vi "ADC SNR_ref_sweep.vi"(8 "error in (no error)":errorcluster, 9 "Sequence parameters":string[][](array[string])=[["Min limit", "Max limit", "Register sheet file", "Register Sheet"], ["", "", "CC2600.xls", "TX_BLE;Trim"], ["Reg write (addr;value)", "Operating frequency [Hz]", "", ""], ["NA", "2.44G", "", ""]], 10 "Run type":i32, 11 "Method parameters":T3={"Dev"={"Do not disturb DUT"=FALSE, "XOSC"=32000000.0, "Board type"="", "EM"="", "Configure tempboard"=TRUE, "Device specific info"=[], "Generic Object"=refnum}, "Method"={"Run type"=1, "Test name"="Current LPM2 4", "Comment"="", "Results folder"="", "AFC"=enum."Off", "Method name"="Current LPM2 4", "Method results"={"Excel brief report"=FALSE, "Spotfire report"=FALSE, "Starfish report"=FALSE}, "Operator"="", "Reference time"=timestamp(0 s since 1904-01-01), "AFC delay"=0.0, "Initialization"=enum."Enabled", "MD5 Sum"="", "HW addon board"=enum."None", "AFC Regsheet"="", "AFC Regfile"=path "", "dummy"=0.0}, "Inst"={"Instr"={"PS1"={"Name"="", "GPIB address"="", "VISA session"=""}, "PS2"={"Name"="", "GPIB address"="", "VISA session"=""}, "TC1"={"Name"="", "GPIB address"="", "VISA session"=""}, "TC2"={"Name"="", "GPIB address"="", "VISA session"=""}, "SA1"={"Name"="", "GPIB address"="", "VISA session"=""}, "SA2"={"Name"="", "GPIB address"="", "VISA session"=""}, "SG1"={"Name"="", "GPIB address"="", "VISA session"=""}, "SG2"={"Name"="", "GPIB address"="", "VISA session"=""}, "SG3"={"Name"="", "GPIB address"="", "VISA session"=""}, "MI1"={"Name"="", "GPIB address"="", "VISA session"=""}, "MI2"={"Name"="", "GPIB address"="", "VISA session"=""}, "SW SA"={"Name"="", "Controller addr"=""}, "SW SG"={"Name"="", "Controller addr"=""}, "MI3"={"Name"="", "GPIB address"="", "VISA session"=""}}, "Switchbox"={"RF Path"=0, "Cal compensation"=enum."TX", "Switchbox gain mode"="", "State"=enum."TX"}, "Instr to control (i.e. SA1)"="Default", "Intrument info string"=""}, "Sequence parameters"=[["Weight", "Min Limit", "Max Limit", "Register Sheet", "", "", "", "", "", "", "", "", ""], ["Vital", "", "1", "LPM2", "", "", "", "", "", "", "", "", ""], ["Resolution", "Reg write (addr;value)", "Chip mode", "Range", "", "", "", "", "", "", "", "", ""], ["u", "NA", "", "auto", "", "", "", "", "", "", "", "", ""]], "Cond"={"Temp logged"=25.0, "VDD1_PS1_6V"=-999.0, "VDD2_PS1_25V"=-999.0, "VDD4_PS2_25V"=-999.0, "VDD3_PS2_6V"=-999.0}, "Meas config"={"X-axis inner loop index"=32000000, "Y-axis outer loop index"=32000000, "X-axis"=[], "Y-axis"=[], "X-axis array req size"=32000000, "Y-axis array req size"=32000000, "Param description"=[], "Use meas clust for reporting"=FALSE, "Parameter index (page)"=0, "X-axis name"="", "Y-axis name"=""}} {"Cond"."VDD3_PS2_6V" format="%.3f"; "Cond"."VDD4_PS2_25V" format="%.3f"; "Cond"."VDD2_PS1_25V" format="%.3f"; "Cond"."VDD1_PS1_6V" format="%.3f"; "Method"."dummy" format="%.1p"; "Method"."AFC delay" format="%.1p"; "Dev"."XOSC" format="%.3p"}) -> (0 "error out":errorcluster, 1 "End method error":T2, 2 "Short Results":string[](array[string])=["0.00", "0.00", "0.00", "0.00"], 3 "Result summary":string[][](array[string])=[["Critical", "Output Power@2405 MHz", "-3", "4", "dBm"], ["Critical", "Output Power@2410 MHz", "-3", "4", "dBm"]])   [LabVIEW 2019]
doc: "[AutoDocStart]Performs crystal accuracy measurements. Measures the offset from ideal frequency. Primarily used for tuning XOSC capacitors and verifying XOSC trims.\n\nSweeping parameters: operating frequency, OSC override value and VDDR level\n\nResults: Offset frequency in ppm[AutoDocEnd]"
uses:
  User Lib/Utilities/Cluster definitions/Method input.ctl
  User Lib/Utilities/Cluster definitions/Device specific info.ctl
  User Lib/Utilities/Controls/Automatic Frequency Compensation types.ctl
  User Lib/Utilities/Controls/Method Reports.ctl
  User Lib/Utilities/Cluster definitions/Method Initialization.ctl
  User Lib/Utilities/Controls/HW addon boards.ctl
  User Lib/Utilities/Cluster definitions/Instr clust.ctl
  User Lib/Utilities/Switchbox control/SwitchBox_State._ENUMctl.ctl
  User Lib/Utilities/Cluster definitions/End method error cluster.ctl
  User Lib/Utilities/Cluster definitions/DUT vdd control.ctl
  User Lib/Utilities/Cluster definitions/DUT VDD4.ctl
  User Lib/Utilities/Cluster definitions/DUT VDD3.ctl
  User Lib/Utilities/Cluster definitions/DUT VDD2.ctl
  User Lib/Utilities/Cluster definitions/DUT VDD1.ctl
  3a26386c-adf8-4bfd-9313-23d3b8777f38.vi
  00a85a70-9fe7-4572-b3d9-e5ce3378243e.vi
  50564926-5797-4515-82f7-8b24a758fedb.vi
  ff8123cc-dee3-4505-8a81-37fe2d556b47.vi
  fd6c0d4b-9dc8-492c-9bac-41f6ad4bdd39.vi
  153c9ed0-a16e-46e5-8e4c-c1ec3d6952ee.vi
  ce3ff4de-b0d2-4c44-a033-17b5da13a9db.vi
  5ebeeef5-e7a0-4ee6-8b8c-49cd29034619.vi
  9df8e1df-3a4c-4a82-932f-cd734a2f5e31.vi
panel:
  in  "Tab Control":T1(tab)
  # "°C"
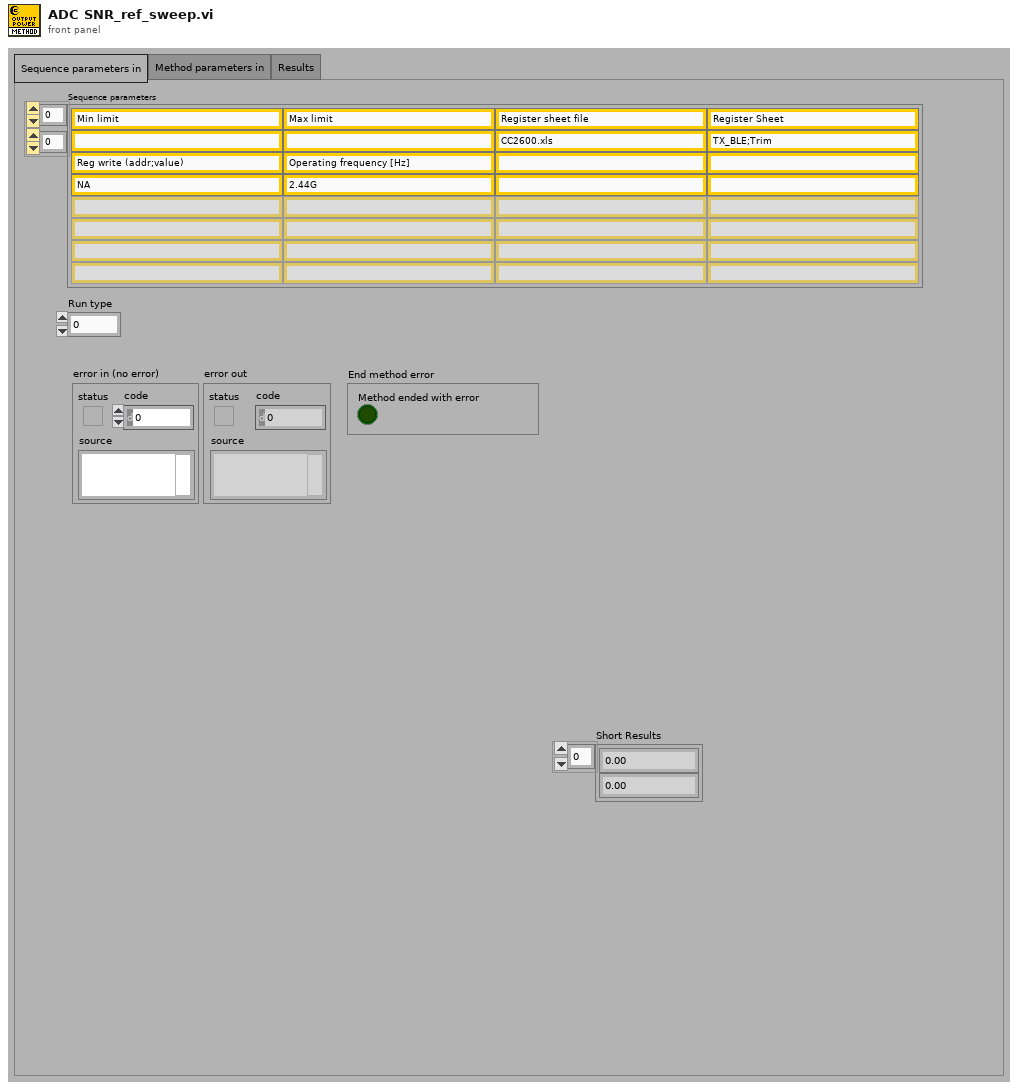
[diagram p1: front panel]
types:
  T1 = enum32{"Sequence parameters in", "Method parameters in", "Results"}
  T2 = typedef "End method error cluster.ctl" = cluster{"Method ended with error":bool}
  T3 = typedef "Method input.ctl" = cluster{"Dev":cluster{"Do not disturb DUT":bool, "XOSC":dbl, "Board type":string, "EM":string, "Configure tempboard":bool, "Device specific info":T4[], "Generic Object":refnum<class>}, "Method":cluster{"Run type":i32, "Test name":string, "Comment":string, "Results folder":string, "AFC":T5, "Method name":string, "Method results":T6, "Operator":string, "Reference time":timestamp, "AFC delay":dbl, "Initialization":T7, "MD5 Sum":string, "HW addon board":T8, "AFC Regsheet":string, "AFC Regfile":path, "dummy":dbl}, "Inst":T9, "Sequence parameters":string[][], "Cond":cluster{"Temp logged":dbl, "VDD1_PS1_6V":dbl, "VDD2_PS1_25V":dbl, "VDD4_PS2_25V":dbl, "VDD3_PS2_6V":dbl}, "Meas config":cluster{"X-axis inner loop index":i32, "Y-axis outer loop index":i32, "X-axis":string[], "Y-axis":string[], "X-axis array req size":i32, "Y-axis array req size":i32, "Param description":string[][], "Use meas clust for reporting":bool, "Parameter index (page)":i32, "X-axis name":string, "Y-axis name":string}}
  T4 = typedef "Device specific info.ctl" = cluster{"EM number":u8, "IP address":string, "Enabled":bool, "Slot no":u8, "RF path":u8, "EM name":string, "Wafer info":string, "AFC frequency ppm":dbl, "Register writes":string[][], "Meas data":string[][][], "Device comment":string}
  T5 = typedef "Automatic Frequency Compensation types.ctl" = enum16{"Off", "Compensate Instrument frequency", "Compensate DUT frequency", "Predictive - Compensate Instrument frequency", "Predictive - Compensate DUT frequency", "Do not skip re-init - Compensate Instrument frequency", "Do not skip re-init - Compensate DUT frequency"}
  T6 = typedef "Method Reports.ctl" = cluster{"Excel brief report":bool, "Spotfire report":bool, "Starfish report":bool}
  T7 = typedef "Method Initialization.ctl" = enum16{"Enabled", "Skip Instr and Device Init", "Enabled with Separate Flash", "Set PS, Device Init and Skip Instr Init", "Skip Device Init"}
  T8 = typedef "HW addon boards.ctl" = enum16{"None", "Current meas 5EM", "Stresstest 10EM"}
  T9 = typedef "Instr clust.ctl" = cluster{"Instr":cluster{"PS1":cluster{"Name":string, "GPIB address":string, "VISA session":refnum<visa-resource-name>}, "PS2":cluster{"Name":string, "GPIB address":string, "VISA session":refnum<visa-resource-name>}, "TC1":cluster{"Name":string, "GPIB address":string, "VISA session":refnum<visa-resource-name>}, "TC2":cluster{"Name":string, "GPIB address":string, "VISA session":refnum<visa-resource-name>}, "SA1":cluster{"Name":string, "GPIB address":string, "VISA session":refnum<visa-resource-name>}, "SA2":cluster{"Name":string, "GPIB address":string, "VISA session":refnum<visa-resource-name>}, "SG1":cluster{"Name":string, "GPIB address":string, "VISA session":refnum<visa-resource-name>}, "SG2":cluster{"Name":string, "GPIB address":string, "VISA session":refnum<visa-resource-name>}, "SG3":cluster{"Name":string, "GPIB address":string, "VISA session":refnum<visa-resource-name>}, "MI1":cluster{"Name":string, "GPIB address":string, "VISA session":refnum<visa-resource-name>}, "MI2":cluster{"Name":string, "GPIB address":string, "VISA session":refnum<visa-resource-name>}, "SW SA":cluster{"Name":string, "Controller addr":string}, "SW SG":cluster{"Name":string, "Controller addr":string}, "MI3":cluster{"Name":string, "GPIB address":string, "VISA session":refnum<visa-resource-name>}}, "Switchbox":cluster{"RF Path":i32, "Cal compensation":enum16{"TX", "RX", "Interferer", "No compensation", "Interferer2"}, "Switchbox gain mode":string, "State":T10}, "Instr to control (i.e. SA1)":string, "Intrument info string":string}
  T10 = typedef "SwitchBox_State._ENUMctl.ctl" = enum16{"TX", "RX", "SP:TX", "SP:RX", "SW:TX", "SW:RX"}
  T11 = typedef "DUT vdd control.ctl" = cluster{"VDD4 config":T12, "VDD3 config":T13, "VDD2 config":T14, "VDD1 config":T15}
  T12 = typedef "DUT VDD4.ctl" = u16
  T13 = typedef "DUT VDD3.ctl" = u16
  T14 = typedef "DUT VDD2.ctl" = u16
  T15 = typedef "DUT VDD1.ctl" = u16
  T16 = cluster{"Fundamental Frequency":dbl, "Sampling Frequncy":dbl, "No of Harmonics":u8, "Window":enum16{"None ", "Hanning", "Hamming", "Blackman-Harris", "Exact Blackman", "Blackman", "Flat Top", "4 Term B-Harris ", "7 Term B-Harris"}, "Blackman (fundamental power) bins)":dbl}
  T17 = enum32{"NI Card Settings", "Memory Read Setting", "DC Capture", "ADC Ramp", "ADC Sine", "SNR", "Cap Calibration"}
  T18 = enum32{"Read from Memory", "Read .dat file", "NI Card Capture", "None"}
  T19 = cluster{"Path to Save plot":path, "Path to Raw Data plot":path}
  T20 = cluster{"Save INL/DNL Plot(Ramp)":bool, "Save SNR Plot":bool, "Save INL/DNL Plot(Sine)":bool, "Save INL/DNL Raw Data(Ramp)":bool, "Save SNR Raw Data":bool, "Save INL/DNL Raw Data(Sine)":bool, "Save DC Raw data":bool, "Save  Raw Data(Sine)":bool}
  T21 = cluster{"SNR":dbl, "SNRD":dbl, "THD":dbl, "ENOB (SNRD)":dbl, "SFDR":dbl, "ENOB (SNR)":dbl, "Noise Power":dbl, "Signal power":dbl}
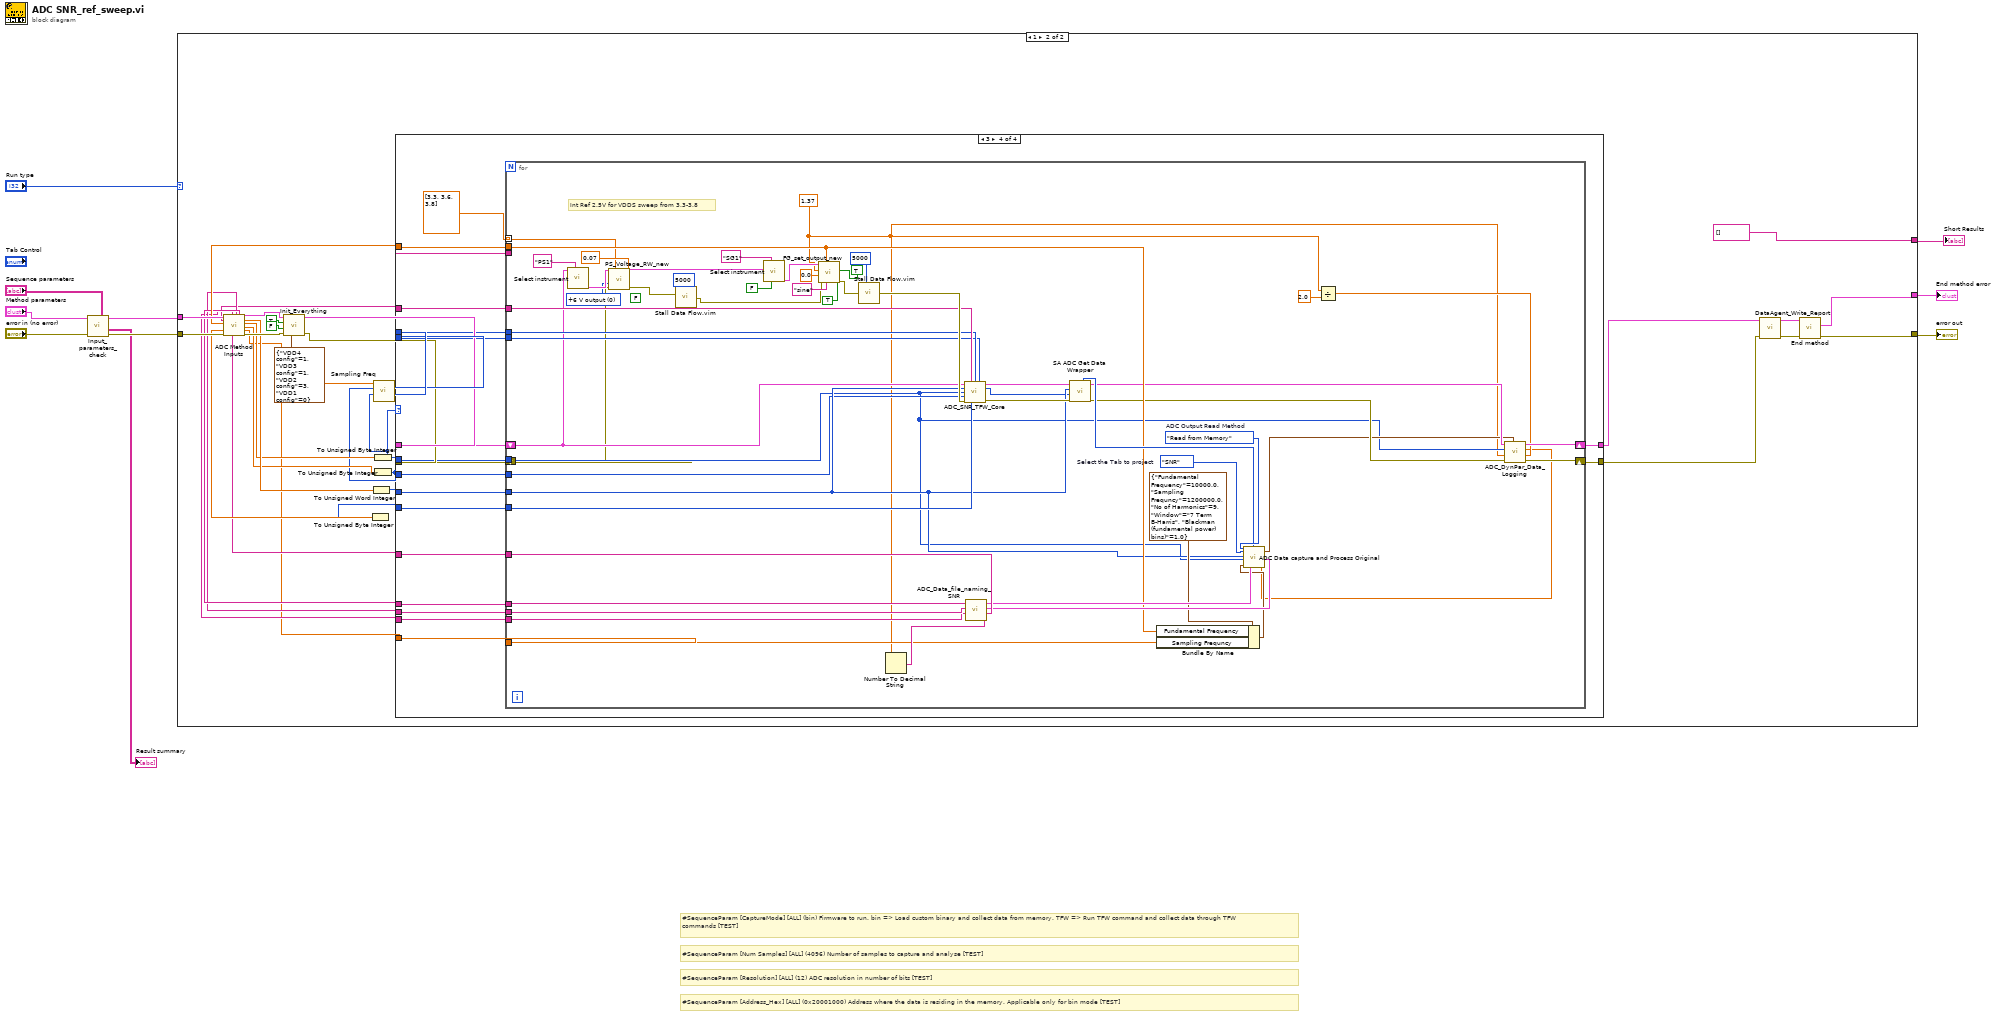
[diagram p0: block diagram]
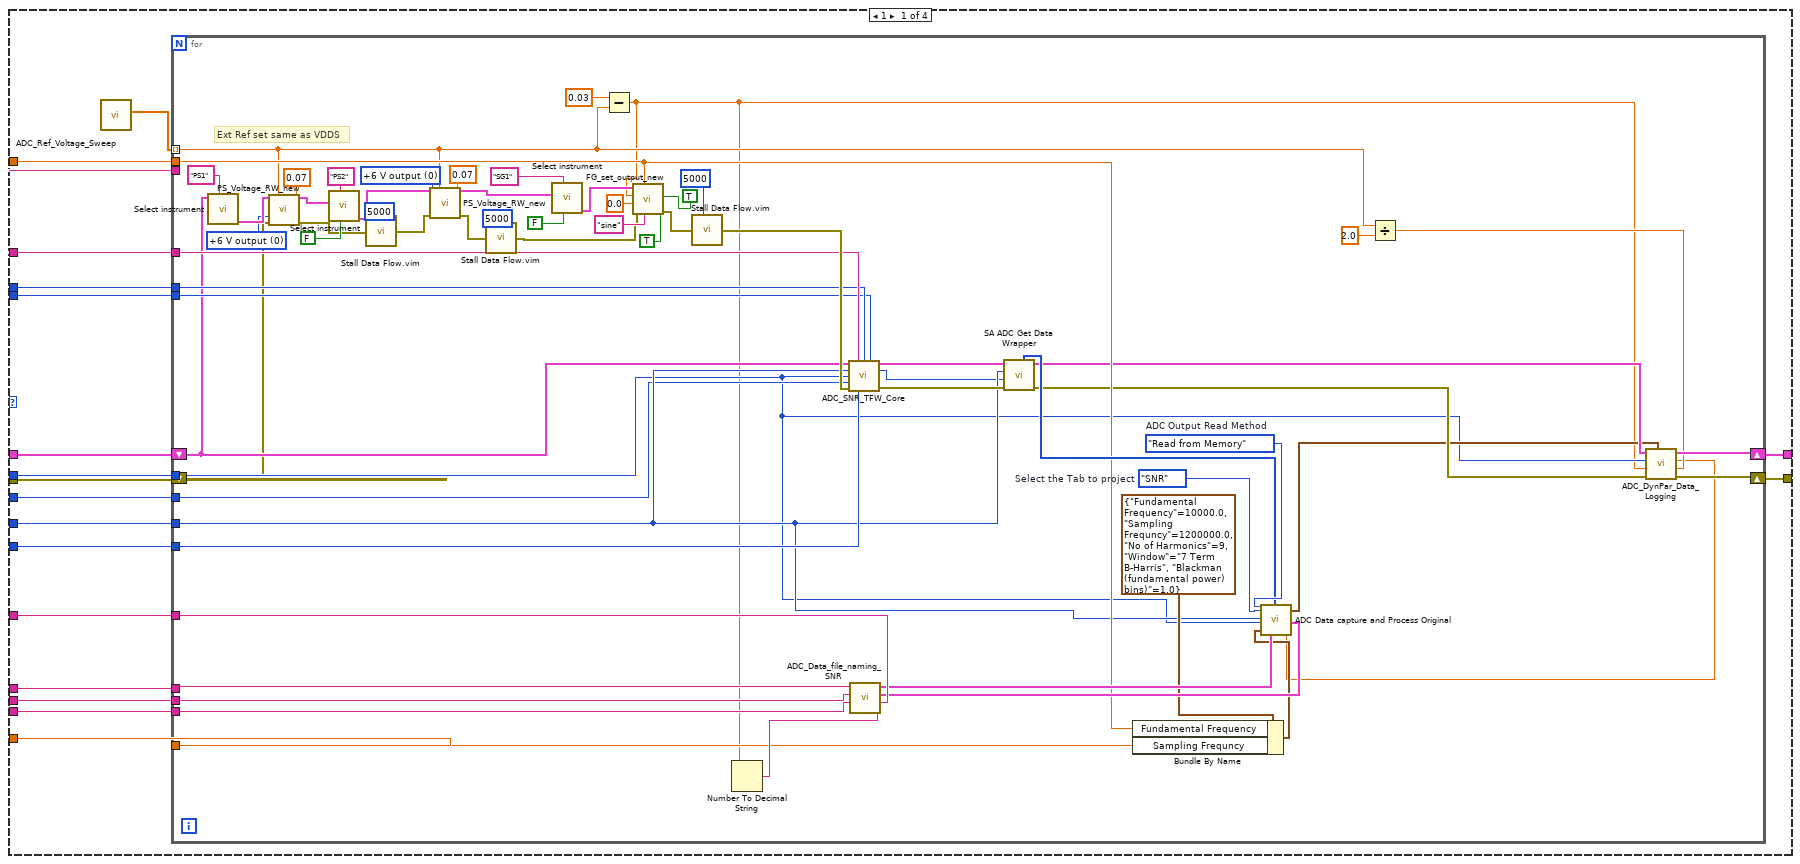
[diagram p3: hidden frame]
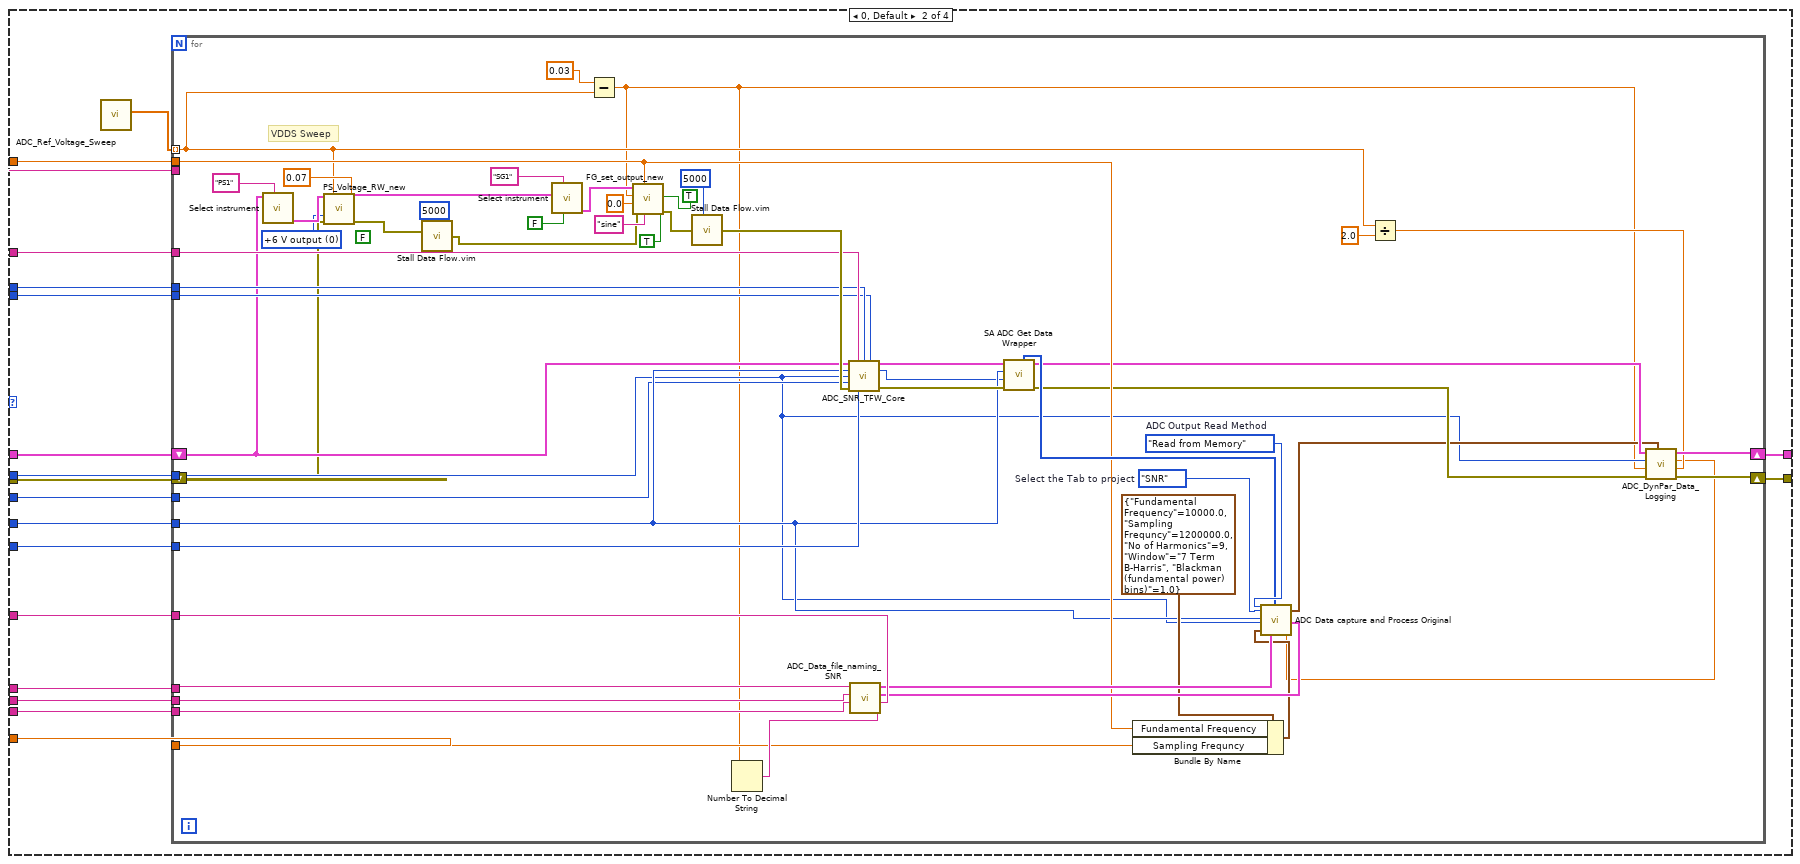
[diagram p4: hidden frame]
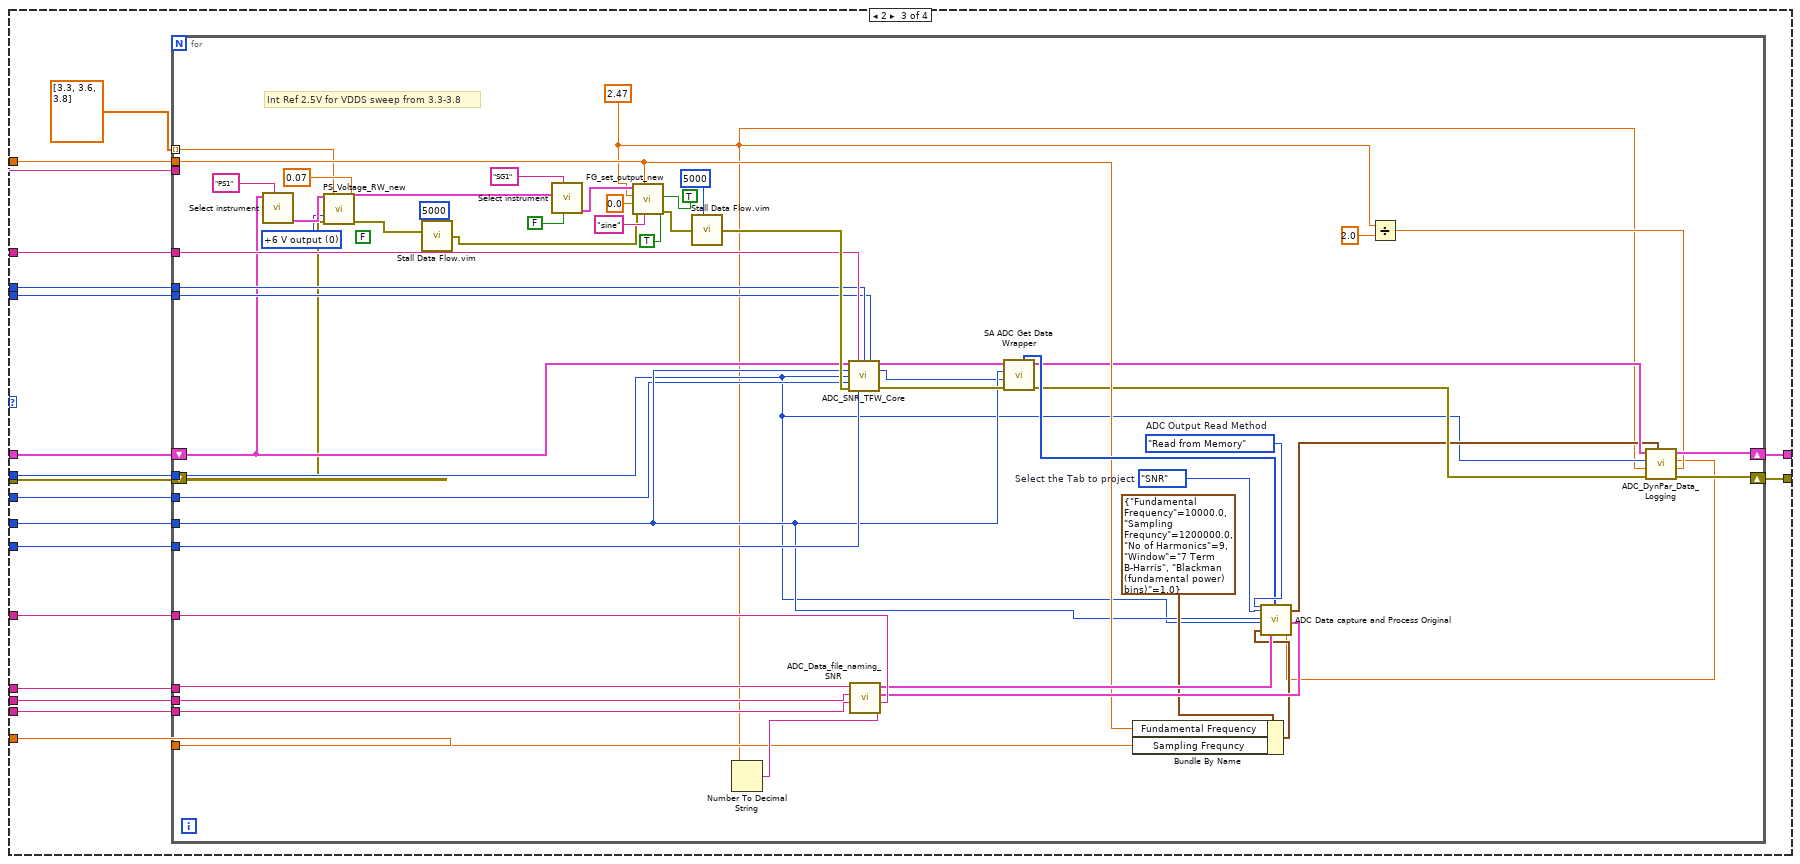
[diagram p5: hidden frame]
diagram:
  # "#SequenceParam [Num Samples] [ALL] (4096) Number of samples to capture and analyse [TEST]"
  # "#SequenceParam [CaptureMode] [ALL] (bin) Firmware to run. bin => Load custom binary and collect data from memory. TFW => Run TFW command and collect data through TFW commands [TEST]"
  # "#SequenceParam [Address_Hex] [ALL] (0x20001000) Address where the data is residing in the memory. Applicable only for bin mode [TEST]"
  # "#SequenceParam [Resolution] [ALL] (12) ADC resolution in number of bits [TEST]"
  n1 = call "Input_parameters_check.vi"("Sequence parameters"="Sequence parameters", "error in"="error in (no error)", "Method cluster in"="Method parameters") -> ("error out"=w9:errorcluster, "Result summary"=→"Result summary":string[][], "Method cluster out"=w5:T3)  [unwired: 6 in]
  n2 = case shown="1" "Run type" {
    tunnel: w9 -> [w11 w33]
    tunnel: [w11 w44] -> w10
    tunnel: w5 -> [_ w34]
    tunnel: [_ w43] -> w4
    tunnel: [_ string[] []] -> w1
    frame 0, Default {
      # "Run type 0 is only for formatting the result summary"
    }
    frame 1 {
      n3 = call "ADC Method Inputs.vi"("Method cluster in"=w34, "error in (no error)"=w33) -> ("Capture Mode"=w16:string, "Signal Freq"=w22:dbl, "ADC Chnl No."=w27:dbl, "Sampling Freq String"=w19:string, "Chnl No. string"=w18:string, "Resolution String"=w20:string, "Voltage Ref String"=w21:string, "Method cluster out"=w31:T3, "Num Samples"=w30:dbl, "Resolution"=w29:dbl, "Voltage Ref"=w28:dbl, "Sampling Freq"=w17:dbl, "error out"=w32:errorcluster)  [unwired: 3 in, 2 out]
      n4 = call "Init_Everything.vi"("VDD config"=T11 {"VDD4 config"=1, "VDD3 config"=1, "VDD2 config"=3, "VDD1 config"=0}, "error in"=w32, "Support current measurement?"=FALSE, "Override VDD Config"=TRUE, "Method cluster In"=w31) -> ("error out"=w12:errorcluster, "Method cluster out"=w13:T3)  [unwired: 3 in, 2 out]
      n5 = To Unsigned Byte Integer(number=w27) -> (unsigned 8bit integer=w25:u8)
      n6 = To Unsigned Word Integer(number=w30) -> (unsigned 16bit integer=w26:u16)
      n7 = To Unsigned Byte Integer(number=w29) -> (unsigned 8bit integer=w14:u8)
      n8 = To Unsigned Byte Integer(number=w28) -> (unsigned 8bit integer=w15:u8)
      n9 = call "Sampling Freq.vi"("Resolution"=w14, "Voltage Ref"=w15, "Sampling Freq"=w17) -> ("LGPT Count"=w24:u16, "SCOMP"=w23:u16)  [unwired: 7 in]
      n10 = case shown="3" w14 {
        tunnel: [w62 w144 w217 w289] -> w38
        tunnel: [w61 w143 w216 w288] -> w37
        tunnel: w26 -> [w60 w142 w215 w287]
        tunnel: w25 -> [w59 w141 w214 w286]
        tunnel: w24 -> [w58 w140 w213 w285]
        tunnel: w23 -> [w57 w139 w212 w284]
        tunnel: w22 -> [w56 w138 w211 w283]
        tunnel: w21 -> [w55 w137 w210 w282]
        tunnel: w20 -> [w54 w136 w209 w281]
        tunnel: w19 -> [w53 w135 w208 w280]
        tunnel: w18 -> [w52 w134 w207 w279]
        tunnel: w17 -> [w51 w133 w206 w278]
        tunnel: w16 -> [w50 w132 w205 w277]
        tunnel: w13 -> [w49 w131 w204 w276]
        tunnel: w12 -> [w48 w130 w203 w275]
        tunnel: w14 -> [w47 w129 w202 w274]
        tunnel: w15 -> [w46 w128 w201 w273]
        frame 1 {
          n11 = call "ADC_Ref_Voltage_Sweep.vi"() -> ("Ref voltage sweep"=w45:dbl[])  [unwired: 11 in]
          n12 = for {
            tunnel: w60 -> [w100]
            tunnel: w47 -> [w98]
            tunnel: w46 -> [w99]
            tunnel: w59 -> [w101]
            tunnel: w50 -> [_]
            tunnel: w58 -> [w96]
            tunnel: w57 -> [w95]
            shift-right: [w111] -> w62
            shift-left: w49 -> [w84]
            shift-right: [w110] -> w61
            shift-left: w48 -> [w82]
            tunnel: w45 -> [w65] mode=indexing
            tunnel: w56 -> [w113]
            tunnel: w55 -> [w124]
            tunnel: w54 -> [w123]
            tunnel: w53 -> [w122]
            tunnel: w52 -> [w125]
            tunnel: w51 -> [w112]
            tunnel: w50 -> [w97]
            w66 = u16 0 items=["+6 V output", "+25 V output", "-25 V output", "ALL TERM"] ("Output Terminals")
            w81 = u16 0 items=["+6 V output", "+25 V output", "-25 V output", "ALL TERM"] ("Output Terminals")
            w117 = T17."SNR"  # Select the Tab to project
            w118 = T18."Read from Memory"  # ADC Output Read Method
            # "Ext Ref set same as VDDS"
            n13 = call "Select instrument.vi"("Instr.Instr to control (i.e. SA1)"="PS1", "Method cluster in"=w84) -> ("Instr out"=w83:T9)  [unwired: 7 in, 2 out]
            n14 = call "PS_Voltage_RW_new.vi"("InstrCluster in"=w83, "Set Voltage"=w65, "Current(0)"=0.07, "Output Terminals"=w81, "error in (no error)"=w82) -> ("InstrCluster out"=w79:T9, "error out"=w77:errorcluster)  [unwired: 8 in, 1 out]
            n15 = call "Select instrument.vi"("Method cluster (T) / Instr cluster (F)"=FALSE, "Instr.Instr to control (i.e. SA1)"="PS2", "Instr in"=w79) -> ("Instr out"=w74:T9)  [unwired: 6 in, 2 out]
            n16 = call "Stall Data Flow.vim"("value in"=w77, "milliseconds to wait"=u32 5000) -> ("value out"=w73:errorcluster)  [unwired: 1 out]
            n17 = call "PS_Voltage_RW_new.vi"("InstrCluster in"=w74, "Set Voltage"=w65, "Current(0)"=0.07, "Output Terminals"=w66, "error in (no error)"=w73) -> ("InstrCluster out"=w69:T9, "error out"=w71:errorcluster)  [unwired: 8 in, 1 out]
            n18 = call "Stall Data Flow.vim"("value in"=w71, "milliseconds to wait"=u32 5000) -> ("value out"=w72:errorcluster)  [unwired: 1 out]
            n19 = call "Select instrument.vi"("Method cluster (T) / Instr cluster (F)"=FALSE, "Instr.Instr to control (i.e. SA1)"="SG1", "Instr in"=w69) -> ("Instr out"=w93:T9)  [unwired: 6 in, 2 out]
            n20 = Subtract(x=0.03, y=w65) -> (x-y=w63:dbl)
            n21 = call "FG_set_output_new.vi"("High impedance (T)"=TRUE, "Enable Output?"=TRUE, "Function (DC, Sine, Square, Triangle, Ramp up, Ramp down, Pulse)"="sine", "Frequency [Hz]"=w113, "error in"=w72, "Low voltage"=0.0, "High voltage (or DC)"=w63, "InstrCluster in"=w93) -> ("error out"=w91:errorcluster)  [unwired: 2 in, 1 out]
            n22 = call "Stall Data Flow.vim"("value in"=w91, "milliseconds to wait"=u32 5000) -> ("value out"=w102:errorcluster)  [unwired: 1 out]
            n23 = Number To Decimal String(number=w63) -> (decimal integer string=w119:string)  [unwired: 1 in]
            n24 = call "ADC_SNR_TFW_Core.vi"("Method cluster in"=w84, "Capture Mode"=w97, "LGPT Count"=w96, "SCOMP"=w95, "No. Samples"=w100, "Resolution"=w98, "Voltage Ref"=w99, "error in"=w102, "ADC Chnl No."=w101) -> ("Method cluster out 2"=w104:T3, "ResPar[0] Data Address"=w94:u32, "error out"=w103:errorcluster)  [unwired: 3 in, 1 out]
            n25 = call "ADC_Data_file_naming_SNR.vi"("Amplitude (Vpp)"=w119, "ADC Chn. No"=w125, "Sampling Freq String"=w122, "Resolution String"=w123, "Voltage Ref String"=w124) -> ("path to save"=w120:T19, "Save data"=w121:T20)  [unwired: 5 in]
            n26 = call "SA ADC Get Data Wrapper.vi"("error in"=w103, "Data Address"=w94, "Num Samples"=w100, "Method cluster in"=w104) -> ("error out"=w108:errorcluster, "output cluster"=w109:T3, "ADC samples"=w116:u32[])  [unwired: 2 in, 3 out]
            n27 = Bundle By Name(cluster=T16 {"Fundamental Frequency"=10000.0, "Sampling Frequncy"=1200000.0, "No of Harmonics"=9, "Window"=enum."7 Term B-Harris", "Blackman (fundamental power) bins)"=1.0} ("Inputs for Dyanmic para"), "Fundamental Frequency"=w113, "Sampling Frequncy"=w112) -> (w114:T16)
            n28 = call "ADC Data capture and Process Original.vi"("ADC Output Read Method"=w118, "Select the Tab to project"=w117, "No.of samples(SNR)"=w100, "Resolution"=w98, "Inputs for Dyanmic para"=w114, "Save data"=w121, "Waveform"=w116, "path to save"=w120) -> ("detected Throughput"=w105:dbl, "Dynamic Parameters"=w107:T21)  [unwired: 13 in, 5 out]
            n29 = Divide(x=w65, y=2.0) -> (x/y=w106:dbl)
            n30 = call "ADC_DynPar_Data_Logging.vi"("Offset (V)"=w106, "detected Throughput"=w105, "Dynamic Parameters"=w107, "error in (no error)"=w108, "Amplitude (Vpp)"=w63, "Ref Voltage"=w98, "Method cluster in"=w109) -> ("error out"=w110:errorcluster, "Method cluster out"=w111:T3)  [unwired: 3 in]
          }
        }
        frame 0, Default {
          n31 = call "ADC_Ref_Voltage_Sweep.vi"() -> ("Ref voltage sweep"=w127:dbl[])  [unwired: 11 in]
          n32 = for {
            tunnel: w142 -> [w173]
            tunnel: w129 -> [w171]
            tunnel: w128 -> [w172]
            tunnel: w141 -> [w174]
            tunnel: w132 -> [_]
            tunnel: w140 -> [w169]
            tunnel: w139 -> [w168]
            shift-right: [w184] -> w144
            shift-left: w131 -> [w157]
            shift-right: [w183] -> w143
            shift-left: w130 -> [w155]
            tunnel: w127 -> [w147] mode=indexing
            tunnel: w138 -> [w186]
            tunnel: w137 -> [w197]
            tunnel: w136 -> [w196]
            tunnel: w135 -> [w195]
            tunnel: w134 -> [w198]
            tunnel: w133 -> [w185]
            tunnel: w132 -> [w170]
            (unwired) FALSE ("Method cluster (T) / Instr cluster (F)")
            w154 = u16 0 items=["+6 V output", "+25 V output", "-25 V output", "ALL TERM"] ("Output Terminals")
            w190 = T17."SNR"  # Select the Tab to project
            w191 = T18."Read from Memory"  # ADC Output Read Method
            # "VDDS Sweep"
            n33 = call "Select instrument.vi"("Instr.Instr to control (i.e. SA1)"="PS1", "Method cluster in"=w157) -> ("Instr out"=w156:T9)  [unwired: 7 in, 2 out]
            n34 = call "PS_Voltage_RW_new.vi"("InstrCluster in"=w156, "Set Voltage"=w147, "Current(0)"=0.07, "Output Terminals"=w154, "error in (no error)"=w155) -> ("InstrCluster out"=w148:T9, "error out"=w152:errorcluster)  [unwired: 8 in, 1 out]
            n35 = call "Stall Data Flow.vim"("value in"=w152, "milliseconds to wait"=u32 5000) -> ("value out"=w149:errorcluster)  [unwired: 1 out]
            n36 = call "Select instrument.vi"("Method cluster (T) / Instr cluster (F)"=FALSE, "Instr.Instr to control (i.e. SA1)"="SG1", "Instr in"=w148) -> ("Instr out"=w166:T9)  [unwired: 6 in, 2 out]
            n37 = Subtract(x=0.03, y=w147) -> (x-y=w145:dbl)
            n38 = call "FG_set_output_new.vi"("High impedance (T)"=TRUE, "Enable Output?"=TRUE, "Function (DC, Sine, Square, Triangle, Ramp up, Ramp down, Pulse)"="sine", "Frequency [Hz]"=w186, "error in"=w149, "Low voltage"=0.0, "High voltage (or DC)"=w145, "InstrCluster in"=w166) -> ("error out"=w164:errorcluster)  [unwired: 2 in, 1 out]
            n39 = call "Stall Data Flow.vim"("value in"=w164, "milliseconds to wait"=u32 5000) -> ("value out"=w175:errorcluster)  [unwired: 1 out]
            n40 = Number To Decimal String(number=w145) -> (decimal integer string=w192:string)  [unwired: 1 in]
            n41 = call "ADC_SNR_TFW_Core.vi"("Method cluster in"=w157, "Capture Mode"=w170, "LGPT Count"=w169, "SCOMP"=w168, "No. Samples"=w173, "Resolution"=w171, "Voltage Ref"=w172, "error in"=w175, "ADC Chnl No."=w174) -> ("Method cluster out 2"=w177:T3, "ResPar[0] Data Address"=w167:u32, "error out"=w176:errorcluster)  [unwired: 3 in, 1 out]
            n42 = call "ADC_Data_file_naming_SNR.vi"("Amplitude (Vpp)"=w192, "ADC Chn. No"=w198, "Sampling Freq String"=w195, "Resolution String"=w196, "Voltage Ref String"=w197) -> ("path to save"=w193:T19, "Save data"=w194:T20)  [unwired: 5 in]
            n43 = call "SA ADC Get Data Wrapper.vi"("error in"=w176, "Data Address"=w167, "Num Samples"=w173, "Method cluster in"=w177) -> ("error out"=w181:errorcluster, "output cluster"=w182:T3, "ADC samples"=w189:u32[])  [unwired: 2 in, 3 out]
            n44 = Bundle By Name(cluster=T16 {"Fundamental Frequency"=10000.0, "Sampling Frequncy"=1200000.0, "No of Harmonics"=9, "Window"=enum."7 Term B-Harris", "Blackman (fundamental power) bins)"=1.0} ("Inputs for Dyanmic para"), "Fundamental Frequency"=w186, "Sampling Frequncy"=w185) -> (w187:T16)
            n45 = call "ADC Data capture and Process Original.vi"("ADC Output Read Method"=w191, "Select the Tab to project"=w190, "No.of samples(SNR)"=w173, "Resolution"=w171, "Inputs for Dyanmic para"=w187, "Save data"=w194, "Waveform"=w189, "path to save"=w193) -> ("detected Throughput"=w178:dbl, "Dynamic Parameters"=w180:T21)  [unwired: 13 in, 5 out]
            n46 = Divide(x=w147, y=2.0) -> (x/y=w179:dbl)
            n47 = call "ADC_DynPar_Data_Logging.vi"("Offset (V)"=w179, "detected Throughput"=w178, "Dynamic Parameters"=w180, "error in (no error)"=w181, "Amplitude (Vpp)"=w145, "Ref Voltage"=w171, "Method cluster in"=w182) -> ("error out"=w183:errorcluster, "Method cluster out"=w184:T3)  [unwired: 3 in]
          }
        }
        frame 2 {
          n48 = for {
            tunnel: w215 -> [w245]
            tunnel: w202 -> [w243]
            tunnel: w201 -> [w244]
            tunnel: w214 -> [w246]
            tunnel: w205 -> [_]
            tunnel: w213 -> [w241]
            tunnel: w212 -> [w240]
            shift-right: [w256] -> w217
            shift-left: w204 -> [w229]
            shift-right: [w255] -> w216
            shift-left: w203 -> [w227]
            tunnel: dbl[] [3.3, 3.6, 3.8] -> [w219] mode=indexing
            tunnel: w211 -> [w258]
            tunnel: w210 -> [w269]
            tunnel: w209 -> [w268]
            tunnel: w208 -> [w267]
            tunnel: w207 -> [w270]
            tunnel: w206 -> [w257]
            tunnel: w205 -> [w242]
            w218 = 2.47
            (unwired) FALSE ("Method cluster (T) / Instr cluster (F)")
            w226 = u16 0 items=["+6 V output", "+25 V output", "-25 V output", "ALL TERM"] ("Output Terminals")
            w262 = T17."SNR"  # Select the Tab to project
            w263 = T18."Read from Memory"  # ADC Output Read Method
            # "Int Ref 2.5V for VDDS sweep from 3.3-3.8"
            n49 = call "Select instrument.vi"("Instr.Instr to control (i.e. SA1)"="PS1", "Method cluster in"=w229) -> ("Instr out"=w228:T9)  [unwired: 7 in, 2 out]
            n50 = call "PS_Voltage_RW_new.vi"("InstrCluster in"=w228, "Set Voltage"=w219, "Current(0)"=0.07, "Output Terminals"=w226, "error in (no error)"=w227) -> ("InstrCluster out"=w220:T9, "error out"=w224:errorcluster)  [unwired: 8 in, 1 out]
            n51 = call "Stall Data Flow.vim"("value in"=w224, "milliseconds to wait"=u32 5000) -> ("value out"=w221:errorcluster)  [unwired: 1 out]
            n52 = call "Select instrument.vi"("Method cluster (T) / Instr cluster (F)"=FALSE, "Instr.Instr to control (i.e. SA1)"="SG1", "Instr in"=w220) -> ("Instr out"=w238:T9)  [unwired: 6 in, 2 out]
            n53 = call "FG_set_output_new.vi"("High impedance (T)"=TRUE, "Enable Output?"=TRUE, "Function (DC, Sine, Square, Triangle, Ramp up, Ramp down, Pulse)"="sine", "Frequency [Hz]"=w258, "error in"=w221, "Low voltage"=0.0, "High voltage (or DC)"=w218, "InstrCluster in"=w238) -> ("error out"=w236:errorcluster)  [unwired: 2 in, 1 out]
            n54 = call "Stall Data Flow.vim"("value in"=w236, "milliseconds to wait"=u32 5000) -> ("value out"=w247:errorcluster)  [unwired: 1 out]
            n55 = Number To Decimal String(number=w218) -> (decimal integer string=w264:string)  [unwired: 1 in]
            n56 = call "ADC_SNR_TFW_Core.vi"("Method cluster in"=w229, "Capture Mode"=w242, "LGPT Count"=w241, "SCOMP"=w240, "No. Samples"=w245, "Resolution"=w243, "Voltage Ref"=w244, "error in"=w247, "ADC Chnl No."=w246) -> ("Method cluster out 2"=w249:T3, "ResPar[0] Data Address"=w239:u32, "error out"=w248:errorcluster)  [unwired: 3 in, 1 out]
            n57 = call "ADC_Data_file_naming_SNR.vi"("Amplitude (Vpp)"=w264, "ADC Chn. No"=w270, "Sampling Freq String"=w267, "Resolution String"=w268, "Voltage Ref String"=w269) -> ("path to save"=w265:T19, "Save data"=w266:T20)  [unwired: 5 in]
            n58 = call "SA ADC Get Data Wrapper.vi"("error in"=w248, "Data Address"=w239, "Num Samples"=w245, "Method cluster in"=w249) -> ("error out"=w253:errorcluster, "output cluster"=w254:T3, "ADC samples"=w261:u32[])  [unwired: 2 in, 3 out]
            n59 = Bundle By Name(cluster=T16 {"Fundamental Frequency"=10000.0, "Sampling Frequncy"=1200000.0, "No of Harmonics"=9, "Window"=enum."7 Term B-Harris", "Blackman (fundamental power) bins)"=1.0} ("Inputs for Dyanmic para"), "Fundamental Frequency"=w258, "Sampling Frequncy"=w257) -> (w259:T16)
            n60 = call "ADC Data capture and Process Original.vi"("ADC Output Read Method"=w263, "Select the Tab to project"=w262, "No.of samples(SNR)"=w245, "Resolution"=w243, "Inputs for Dyanmic para"=w259, "Save data"=w266, "Waveform"=w261, "path to save"=w265) -> ("detected Throughput"=w250:dbl, "Dynamic Parameters"=w252:T21)  [unwired: 13 in, 5 out]
            n61 = Divide(x=w218, y=2.0) -> (x/y=w251:dbl)
            n62 = call "ADC_DynPar_Data_Logging.vi"("Offset (V)"=w251, "detected Throughput"=w250, "Dynamic Parameters"=w252, "error in (no error)"=w253, "Amplitude (Vpp)"=w218, "Ref Voltage"=w243, "Method cluster in"=w254) -> ("error out"=w255:errorcluster, "Method cluster out"=w256:T3)  [unwired: 3 in]
          }
        }
        frame 3 {
          n63 = for {
            tunnel: w287 -> [w317]
            tunnel: w274 -> [w315]
            tunnel: w273 -> [w316]
            tunnel: w286 -> [w318]
            tunnel: w277 -> [_]
            tunnel: w285 -> [w313]
            tunnel: w284 -> [w312]
            shift-right: [w328] -> w289
            shift-left: w276 -> [w301]
            shift-right: [w327] -> w288
            shift-left: w275 -> [w299]
            tunnel: dbl[] [3.3, 3.6, 3.8] -> [w291] mode=indexing
            tunnel: w283 -> [w330]
            tunnel: w282 -> [w341]
            tunnel: w281 -> [w340]
            tunnel: w280 -> [w339]
            tunnel: w279 -> [w342]
            tunnel: w278 -> [w329]
            tunnel: w277 -> [w314]
            w290 = 1.37
            (unwired) FALSE ("Method cluster (T) / Instr cluster (F)")
            w298 = u16 0 items=["+6 V output", "+25 V output", "-25 V output", "ALL TERM"] ("Output Terminals")
            w334 = T17."SNR"  # Select the Tab to project
            w335 = T18."Read from Memory"  # ADC Output Read Method
            # "Int Ref 2.5V for VDDS sweep from 3.3-3.8"
            n64 = call "Select instrument.vi"("Instr.Instr to control (i.e. SA1)"="PS1", "Method cluster in"=w301) -> ("Instr out"=w300:T9)  [unwired: 7 in, 2 out]
            n65 = call "PS_Voltage_RW_new.vi"("InstrCluster in"=w300, "Set Voltage"=w291, "Current(0)"=0.07, "Output Terminals"=w298, "error in (no error)"=w299) -> ("InstrCluster out"=w292:T9, "error out"=w296:errorcluster)  [unwired: 8 in, 1 out]
            n66 = call "Stall Data Flow.vim"("value in"=w296, "milliseconds to wait"=u32 5000) -> ("value out"=w293:errorcluster)  [unwired: 1 out]
            n67 = call "Select instrument.vi"("Method cluster (T) / Instr cluster (F)"=FALSE, "Instr.Instr to control (i.e. SA1)"="SG1", "Instr in"=w292) -> ("Instr out"=w310:T9)  [unwired: 6 in, 2 out]
            n68 = call "FG_set_output_new.vi"("High impedance (T)"=TRUE, "Enable Output?"=TRUE, "Function (DC, Sine, Square, Triangle, Ramp up, Ramp down, Pulse)"="sine", "Frequency [Hz]"=w330, "error in"=w293, "Low voltage"=0.0, "High voltage (or DC)"=w290, "InstrCluster in"=w310) -> ("error out"=w308:errorcluster)  [unwired: 2 in, 1 out]
            n69 = call "Stall Data Flow.vim"("value in"=w308, "milliseconds to wait"=u32 5000) -> ("value out"=w319:errorcluster)  [unwired: 1 out]
            n70 = Number To Decimal String(number=w290) -> (decimal integer string=w336:string)  [unwired: 1 in]
            n71 = call "ADC_SNR_TFW_Core.vi"("Method cluster in"=w301, "Capture Mode"=w314, "LGPT Count"=w313, "SCOMP"=w312, "No. Samples"=w317, "Resolution"=w315, "Voltage Ref"=w316, "error in"=w319, "ADC Chnl No."=w318) -> ("Method cluster out 2"=w321:T3, "ResPar[0] Data Address"=w311:u32, "error out"=w320:errorcluster)  [unwired: 3 in, 1 out]
            n72 = call "ADC_Data_file_naming_SNR.vi"("Amplitude (Vpp)"=w336, "ADC Chn. No"=w342, "Sampling Freq String"=w339, "Resolution String"=w340, "Voltage Ref String"=w341) -> ("path to save"=w337:T19, "Save data"=w338:T20)  [unwired: 5 in]
            n73 = call "SA ADC Get Data Wrapper.vi"("error in"=w320, "Data Address"=w311, "Num Samples"=w317, "Method cluster in"=w321) -> ("error out"=w325:errorcluster, "output cluster"=w326:T3, "ADC samples"=w333:u32[])  [unwired: 2 in, 3 out]
            n74 = Bundle By Name(cluster=T16 {"Fundamental Frequency"=10000.0, "Sampling Frequncy"=1200000.0, "No of Harmonics"=9, "Window"=enum."7 Term B-Harris", "Blackman (fundamental power) bins)"=1.0} ("Inputs for Dyanmic para"), "Fundamental Frequency"=w330, "Sampling Frequncy"=w329) -> (w331:T16)
            n75 = call "ADC Data capture and Process Original.vi"("ADC Output Read Method"=w335, "Select the Tab to project"=w334, "No.of samples(SNR)"=w317, "Resolution"=w315, "Inputs for Dyanmic para"=w331, "Save data"=w338, "Waveform"=w333, "path to save"=w337) -> ("detected Throughput"=w322:dbl, "Dynamic Parameters"=w324:T21)  [unwired: 13 in, 5 out]
            n76 = Divide(x=w290, y=2.0) -> (x/y=w323:dbl)
            n77 = call "ADC_DynPar_Data_Logging.vi"("Offset (V)"=w323, "detected Throughput"=w322, "Dynamic Parameters"=w324, "error in (no error)"=w325, "Amplitude (Vpp)"=w290, "Ref Voltage"=w315, "Method cluster in"=w326) -> ("error out"=w327:errorcluster, "Method cluster out"=w328:T3)  [unwired: 3 in]
          }
        }
      }
      n78 = call "DataAgent_Write_Report.vi"("error in (no error)"=w37, "Method cluster in"=w38) -> ("error out"=w41:errorcluster, "Method cluster out"=w40:T3)  [unwired: 8 in]
      n79 = call "End method.vi"("error in"=w41, "Method cluster in"=w40) -> ("error out"=w44:errorcluster, "End method error"=w43:T2)  [unwired: 7 in, 1 out]
    }
  }
  "error out" <- w10
  "End method error" <- w4
  "Short Results" <- w1
